vi "Read Data from 256-bit FIFO.vi"(7 "FIFO In":refnum<k21>="ContinuousInputStream", 9 "Get New Data?":bool) -> (1 "Data Valid":bool, 2 "FIFO Data":i16[](array[numeric]))   [LabVIEW 2011]
uses:
  <vilib>/rvi/DataTransferAndStorage/Container/Common/niFpgaContainerExecOnDevCompGetState.vi
  <vilib>/rvi/FIFO/Fifo_Resource/nirvififoEmulationSetSize.vi
  <vilib>/rvi/DataTransferAndStorage/Container/Common/niFpgaContainerGetUniqueNameForEmu.vi
  <vilib>/rvi/interface/RandomDataEmulation/nirviRandomDataFPGAFIFO.vi
  <vilib>/rvi/interface/RandomDataEmulation/niFpgaRandomDataHandleErrors.vi
  <vilib>/rvi/eio/common/nirviEmuReportErrorAndStop.vi
  <vilib>/rvi/DataTransferAndStorage/Container/XNode/niFpgaContainer.xnode
  <vilib>/rvi/FIFO/Fifo_Resource/niFpgaFifoEmulationRefIn.vi
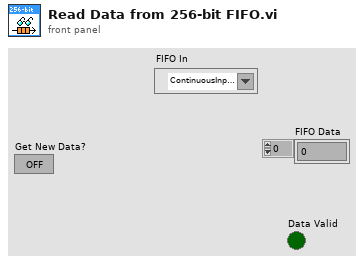
[diagram p1: front panel]
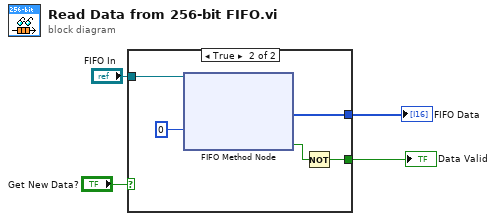
[diagram p0: block diagram]
diagram:
  n1 = case shown="True" "Get New Data?" {
    tunnel: "FIFO In" -> [_ w9]
    tunnel: [_ w7] -> w3
    tunnel: [_ w5] -> w1
    frame False {
    }
    frame True {
      n2 = xnode ("FIFO Method Node")("Timeout"=0, "FIFO In"=w9) -> ("Element"=w7:i16[], "Timed Out?"=w6:bool)  [unwired: 1 out]
      n3 = Not(x=w6) -> (.not. x?=w5:bool)
    }
  }
  "FIFO Data" <- w3
  "Data Valid" <- w1
